vi "COMinput.vi"() -> ()   [LabVIEW 2014]
uses:
  <vilib>/Instr/_visa.llb/VISA Set IO Buffer Mask.ctl
  <vilib>/Instr/_visa.llb/VISA Configure Serial Port (Instr).vi
panel:
  out "error out":errorcluster
  in  "stop":bool
  in  "size (4096)":u32
  in  "Mask":T1=16 items=["I/O Receive Buffer"=16, "I/O Transmit Buffer"=32, "I/O Receive and Transmit Buffer"=48]
  in  "baud rate":u32=115200
  in  "data bits (8)":u16=8
  in  "parity (0:none)":enum16{"None", "Odd", "Even", "Mark", "Space"}(ring)
  in  "VISA resource name":refnum<visa-resource-name>
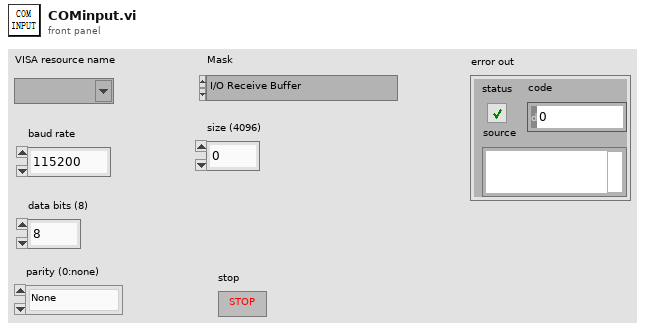
[diagram p1: front panel]
types:
  T1 = typedef "VISA Set IO Buffer Mask.ctl" = u16
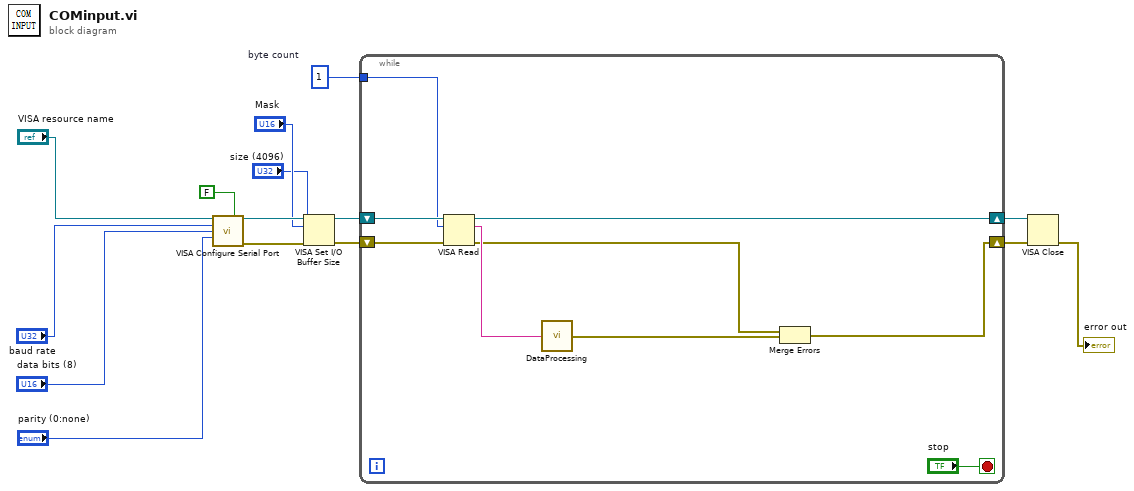
[diagram p0: block diagram]
diagram:
  w2 = u32 1  # byte count
  n1 = call-poly "VISA Configure Serial Port"("VISA resource name"="VISA resource name", "Enable Termination\nChar (T)"=FALSE ("Enable Termination\nChar (T)"), "baud rate (9600)"="baud rate", "data bits (8)"="data bits (8)", "parity (0:none)"="parity (0:none)") -> ("VISA resource name out"=w10:refnum<visa-resource-name>, "error out"=w9:errorcluster)  [unwired: 9 in]
  n2 = VISA Set I/O Buffer Size(VISA resource name=w10, mask (16)="Mask", size (4096)="size (4096)", error in (no error)=w9) -> (VISA resource name out=w6:refnum<visa-resource-name>, error out=w5:errorcluster)
  n3 = while {
    shift-right: [w24] -> w8
    shift-left: w6 -> [w23]
    shift-right: [w16] -> w7
    shift-left: w5 -> [w22]
    tunnel: w2 -> [w21]
    stop <- "stop" stop-if-true
    n4 = VISA Read(VISA resource name=w23, byte count=w21, error in (no error)=w22) -> (VISA resource name out=w24:refnum<visa-resource-name>, read buffer=w19:string, error out=w17:errorcluster)  [unwired: 1 out]
    n5 = call "DataProcessing.vi"("read buffer"=w19) -> ("error out"=w18:errorcluster)
    n6 = Merge Errors(w17, w18) -> (w16:errorcluster)
  }
  n7 = VISA Close(VISA resource name=w8, error in (no error)=w7) -> (error out=→"error out":errorcluster)
